vi "BasicArray.vi"() -> ()   [LabVIEW 2016, in "DronaTest.lvlib" / "test_ValueSignal.lvlib"]
uses:
  test_ValueSignal.lvlib
  main/apis/Setup/GetVI/GetVIByPath.vi
  main/apis/Stimulus/ValueSignal/ValueSignalByPathString.vi
  main/apis/Assert/AssertControlValue/Equal.vi
  <vilib>/addons/_JKI Toolkits/Caraya/classes/Test/Test.lvclass
  main/Drona.lvlib
  main/apis/Stimulus/ValueSignal/ValueSignal.lvlib
  main/apis/Assert/AssertControlValue/AssertControlValue.lvlib
  main/apis/Setup/GetVI/GetVI.lvlib
panel:
  out "error out":errorcluster
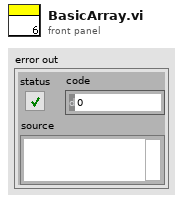
[diagram p1: front panel]
types:
  T1 = cluster{"Numeric":dbl, "String":string, "Boolean":bool}[]
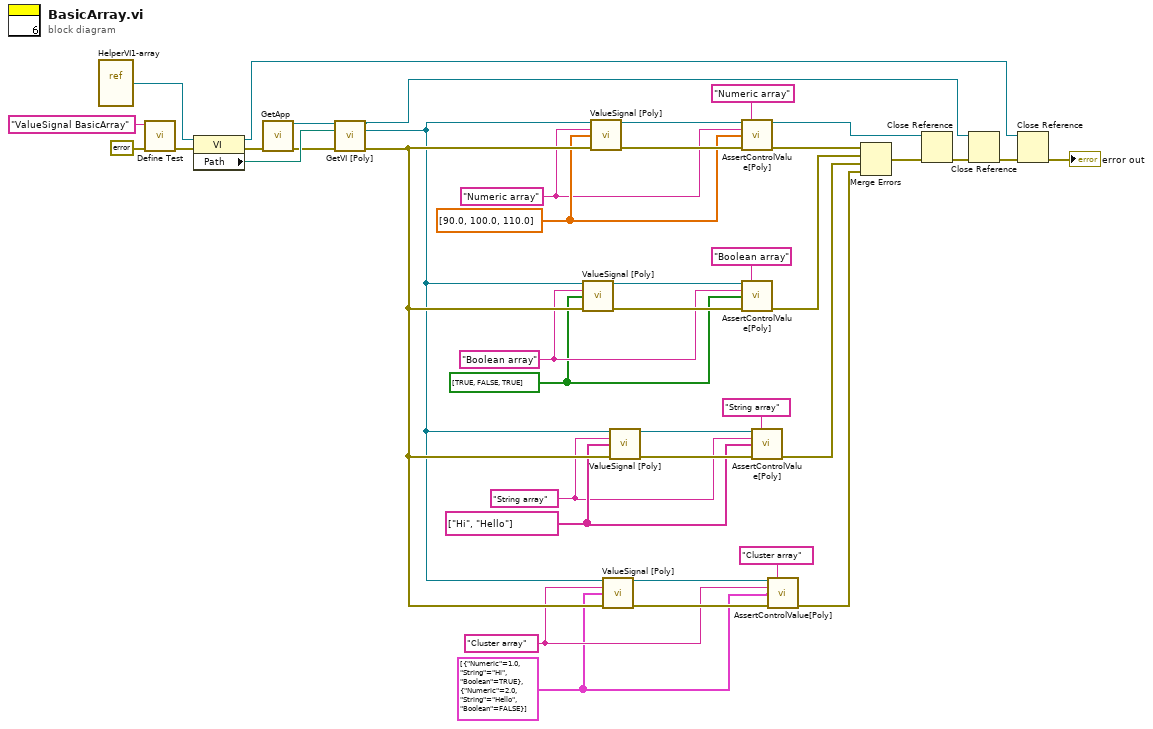
[diagram p0: block diagram]
diagram:
  w2 = T1 [{"Numeric"=1.0, "String"="Hi", "Boolean"=TRUE}, {"Numeric"=2.0, "String"="Hello", "Boolean"=FALSE}] ("Cluster array")
  w3 = "Cluster array" ("Class Name")
  w10 = string[] ["Hi", "Hello"]
  w9 = "String array" ("Class Name")
  w13 = bool[] [TRUE, FALSE, TRUE]
  w14 = "Boolean array" ("Class Name")
  w22 = dbl[] [90.0, 100.0, 110.0]
  w21 = "Numeric array" ("Class Name")
  n1 = vi-ref "HelperVI1-array.vi"() -> (w30:refnum<vi>)
  n2 = call <vilib>:"Define Test.vi"("error in (no error)"=errorcluster {"status"=FALSE, "code"=0, "source"=""}, "Label (VI Title)"="ValueSignal BasicArray") -> ("error out"=w32:errorcluster)  [unwired: 9 in]
  n3 = property on="Property Node" class="VI"(reference=w30, error in=w32) -> (reference out=w26:refnum<vi>, error out=w36:errorcluster, "Path"=w35:path)
  n4 = call "GetApp.vi"("error in (no error)"=w36) -> ("Application Ref"=w37:refnum<vi>, "error out"=w34:errorcluster)  [unwired: 13 in]
  n5 = call-poly "GetVI [Poly].vi"("Application Ref in"=w37, "VI Path"=w35, "error in (no error)"=w34) -> ("Application Ref out"=w27:refnum<vi>, "VI Reference"=w28:refnum<vi>, "error out"=w29:errorcluster)  [unwired: 10 in]
  n6 = call-poly "ValueSignal [Poly].vi"("VI Reference In"=w28, "Control Name"=w14, "Value (Signaling)"=w13, "error in"=w29) -> ("VI Reference Out"=w15:refnum<vi>, "error out"=w18:errorcluster)  [unwired: 10 in]
  n7 = call-poly "ValueSignal [Poly].vi"("VI Reference In"=w28, "Control Name"=w21, "Value (Signaling)"=w22, "error in"=w29) -> ("VI Reference Out"=w20:refnum<vi>, "error out"=w24:errorcluster)  [unwired: 10 in]
  n8 = call-poly "ValueSignal [Poly].vi"("VI Reference In"=w28, "Control Name"=w3, "Value (Signaling)"=w2, "error in"=w29) -> ("VI Reference Out"=w4:refnum<vi>, "error out"=w6:errorcluster)  [unwired: 10 in]
  n9 = call-poly "ValueSignal [Poly].vi"("VI Reference In"=w28, "Control Name"=w9, "Value (Signaling)"=w10, "error in"=w29) -> ("VI Reference Out"=w8:refnum<vi>, "error out"=w12:errorcluster)  [unwired: 10 in]
  n10 = call-poly "AssertControlValue[Poly].vi"("VI Reference In"=w20, "Label"="Numeric array" ("Label (VI Title)"), "Control Name"=w21, "Control Value"=w22, "Error In"=w24) -> ("VI Reference Out"=w19:refnum<vi>, "Error Out"=w23:errorcluster)  [unwired: 9 in]
  n11 = call-poly "AssertControlValue[Poly].vi"("VI Reference In"=w15, "Label"="Boolean array" ("Label (VI Title)"), "Control Name"=w14, "Control Value"=w13, "Error In"=w18) -> ("Error Out"=w17:errorcluster)  [unwired: 9 in, 1 out]
  n12 = call-poly "AssertControlValue[Poly].vi"("VI Reference In"=w8, "Label"="String array" ("Label (VI Title)"), "Control Name"=w9, "Control Value"=w10, "Error In"=w12) -> ("Error Out"=w11:errorcluster)  [unwired: 9 in, 1 out]
  n13 = call-poly "AssertControlValue[Poly].vi"("VI Reference In"=w4, "Label"="Cluster array" ("Label (VI Title)"), "Control Name"=w3, "Control Value"=w2, "Error In"=w6) -> ("Error Out"=w5:errorcluster)  [unwired: 9 in, 1 out]
  n14 = Merge Errors(w23, w17, w11, w5) -> (w40:errorcluster)
  n15 = Close Reference(reference=w19, error in (no error)=w40) -> (error out=w39:errorcluster)
  n16 = Close Reference(reference=w27, error in (no error)=w39) -> (error out=w38:errorcluster)
  n17 = Close Reference(reference=w26, error in (no error)=w38) -> (error out=→"error out":errorcluster)
